vi "Motor Control NO PID AE Ver.vi"(0 "Direction":T2, 1 "AE Mode":T1, 2 "Speed":dbl, 3 "error in (no error)":errorcluster, 4 "Yaw":dbl) -> (5 "Speed & distance":T3, 6 "error out":errorcluster)   [LabVIEW 2018]
uses:
  MOTOR CONTROL NO PID AE DIRECTIONS type def.ctl
  MOTOR CONTROL NO PID AE DATA ENTRY MODE Type def.ctl
  <vilib>/Studica/Studica Toolkit/Background/Mxp Selection.ctl
panel:
  out "M2":dbl
  out "M1":dbl
  out "M0":dbl
  out "S2":dbl
  out "S1":dbl
  out "S0":dbl
  out "M2 Distance":dbl
  out "M1 Distance":dbl
  out "M0 Distance":dbl
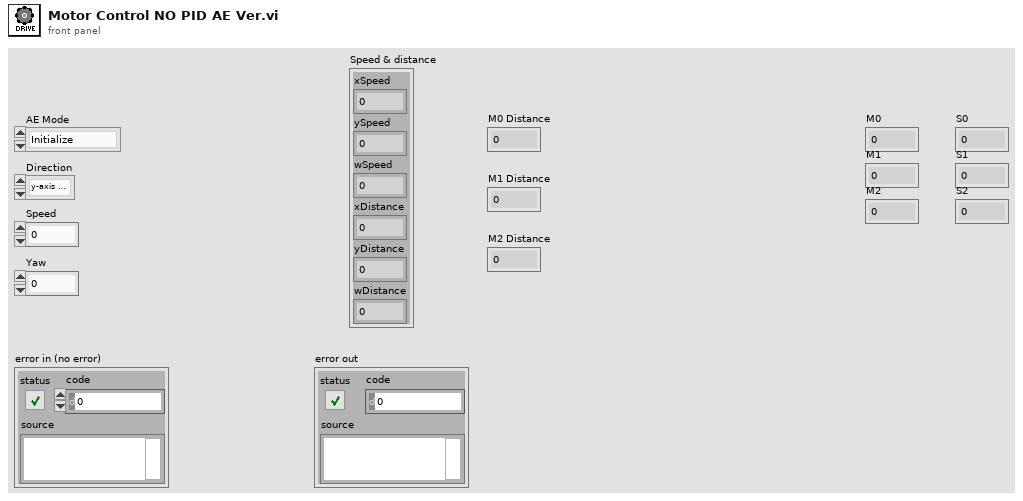
[diagram p1: front panel]
types:
  T1 = typedef "MOTOR CONTROL NO PID AE DATA ENTRY MODE Type def.ctl" = enum16{"Initialize", "Reset Encoders", "Write to motors", "Read from Encoders"}
  T2 = typedef "MOTOR CONTROL NO PID AE DIRECTIONS type def.ctl" = enum16{"y-axis movement", "x-axis movement", "Rotate", "Stop"}
  T3 = cluster{"xSpeed":dbl, "ySpeed":dbl, "wSpeed":dbl, "xDistance":dbl, "yDistance":dbl, "wDistance":dbl}
  T4 = typedef "Mxp Selection.ctl" = enum16{"MXP A", "MXP B"}
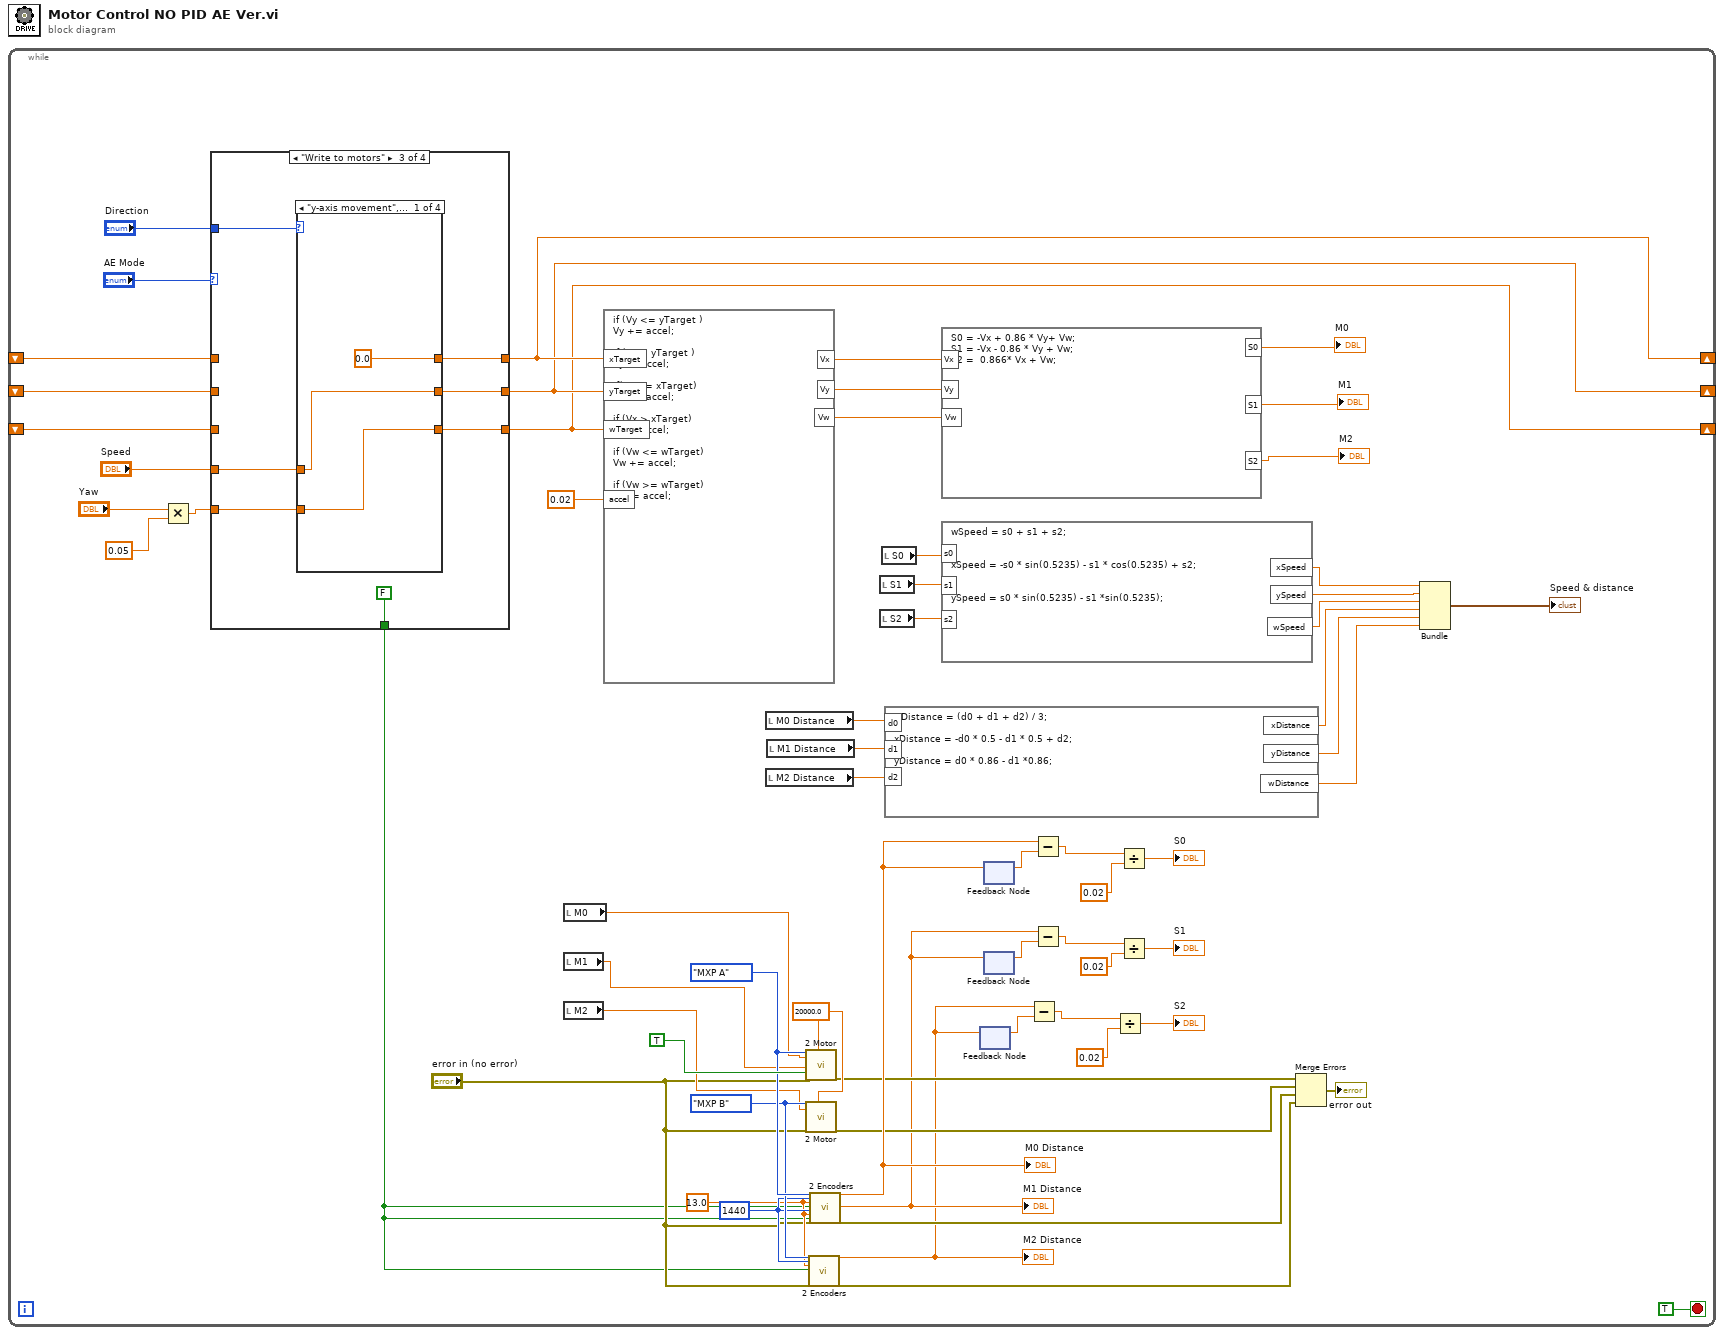
[diagram p0: block diagram]
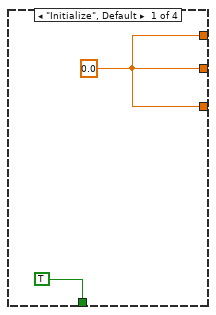
[diagram p2: hidden frame]
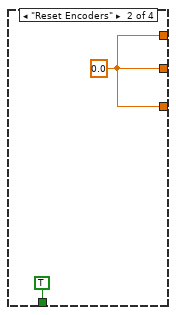
[diagram p3: hidden frame]
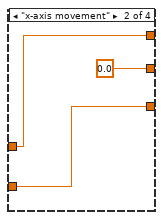
[diagram p4: hidden frame]
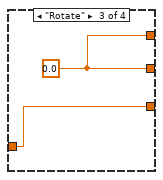
[diagram p5: hidden frame]
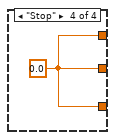
[diagram p6: hidden frame]
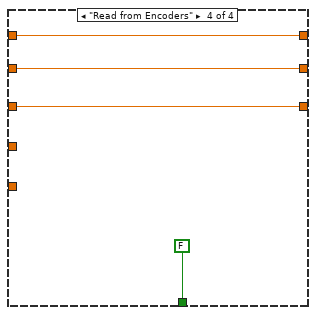
[diagram p7: hidden frame]
diagram:
  n1 = while {
    shift-right: [w11] -> _
    shift-left: _ -> [w7]
    shift-right: [w10] -> _
    shift-left: _ -> [w6]
    shift-right: [w9] -> _
    shift-left: _ -> [w5]
    stop <- TRUE stop-if-true
    w59 = 13.0 ("Wheel Diameter M0 (inches)")
    w60 = u32 1440 ("Ticks Per Rev M0")
    w64 = 20000.0 ("Frequency [Hz]")
    w62 = Mxp_Selection."MXP A" ("Mxp Side")
    w61 = Mxp_Selection."MXP B" ("Mxp Side")
    n2 = Multiply(x="Yaw", y=0.05) -> (x*y=w3:dbl)
    n3 = case shown="\"Write to motors\"" "AE Mode" {
      tunnel: "Direction" -> [_ _ w75 _]
      tunnel: "Speed" -> [_ _ w74 _]
      tunnel: w3 -> [_ _ w73 _]
      tunnel: [w66 w67 w72 w88] -> w11
      tunnel: [w66 w67 w71 w86] -> w9
      tunnel: [w66 w67 w70 w87] -> w10
      tunnel: w7 -> [_ _ _ w88]
      tunnel: w6 -> [_ _ _ w87]
      tunnel: w5 -> [_ _ _ w86]
      tunnel: [TRUE TRUE FALSE FALSE] -> w4
      frame "Initialize", Default {
        w66 = 0.0 ("input variable")
      }
      frame "Reset Encoders" {
        w67 = 0.0 ("input variable")
      }
      frame "Write to motors" {
        n4 = case shown="\"y-axis movement\", Default" w75 {
          tunnel: w74 -> [w78 w81 w83 _]
          tunnel: w73 -> [w77 w80 _ _]
          tunnel: [0.0 ("Speed") w81 w82 w84] -> w72
          tunnel: [w77 w80 w83 w84] -> w71
          tunnel: [w78 0.0 ("input variable") w82 w84] -> w70
          frame "y-axis movement", Default {
          }
          frame "x-axis movement" {
          }
          frame "Rotate" {
            w82 = 0.0 ("input variable")
          }
          frame "Stop" {
            w84 = 0.0 ("input variable")
          }
        }
      }
      frame "Read from Encoders" {
      }
    }
    n5 = local read "M0"() -> (w38:dbl)
    n6 = local read "M1"() -> (w37:dbl)
    n7 = local read "M2"() -> (w36:dbl)
    n8 = formula code="if (Vy <= yTarget )\nVy += accel;\n\nif (Vy > yTarget )\nVy -= accel;\n\nif(Vx <= xTarget)\nVx += accel;\n\nif (Vx > xTarget)\nVx -= accel;\n\nif (Vw <= wTarget)\nVw += accel;\n\nif (Vw >= wTarget)\nVw -= accel;"("xTarget"=w11, "yTarget"=w10, "wTarget"=w9, "accel"=0.02 ("input variable")) -> ("Vy"=w19:dbl, "Vx"=w20:dbl, "Vw"=w18:dbl)
    n9 = local read "M0 Distance"() -> (w32:dbl)
    n10 = local read "M2 Distance"() -> (w30:dbl)
    n11 = local read "M1 Distance"() -> (w31:dbl)
    n12 = call <vilib>:"2 Motor.vi"("Mxp Side"=w62, "Speed M0"=w38, "Speed M1"=w37, "Invert M1"=TRUE, "error in (no error)"="error in (no error)", "Frequency [Hz]"=w64) -> ("error out"=w54:errorcluster)  [unwired: 13 in]
    n13 = call <vilib>:"2 Motor.vi"("Mxp Side"=w61, "Speed M0"=w36, "error in (no error)"="error in (no error)", "Frequency [Hz]"=w64) -> ("error out"=w53:errorcluster)  [unwired: 15 in]
    n14 = call <vilib>:"2 Encoders.vi"("Mxp Side"=w61, "Ticks Per Rev M0"=w60, "Wheel Diameter M0 (inches)"=w59, "Reset Encoder 0"=w4, "error in (no error)"="error in (no error)") -> ("Distance M0 (inches)"=w42:dbl, "error out"=w51:errorcluster)  [unwired: 20 in, 1 out]
    "M2 Distance" <- w42
    n15 = call <vilib>:"2 Encoders.vi"("Mxp Side"=w62, "Ticks Per Rev M0"=w60, "Wheel Diameter M0 (inches)"=w59, "Reset Encoder 0"=w4, "Ticks Per Rev M1"=w60, "Wheel Diameter M1 (inches)"=w59, "Reset Encoder 1"=w4, "error in (no error)"="error in (no error)") -> ("Distance M0 (inches)"=w57:dbl, "Distance M1 (inches)"=w46:dbl, "error out"=w52:errorcluster)  [unwired: 17 in]
    "M0 Distance" <- w57
    "M1 Distance" <- w46
    n16 = local read "S1"() -> (w34:dbl)
    n17 = local read "S2"() -> (w33:dbl)
    n18 = local read "S0"() -> (w35:dbl)
    n19 = formula code="wDistance = (d0 + d1 + d2) / 3;\n\nxDistance = -d0 * 0.5 - d1 * 0.5 + d2;\n\nyDistance = d0 * 0.86 - d1 *0.86;"("d0"=w32, "d1"=w31, "d2"=w30) -> ("xDistance"=w25:dbl, "wDistance"=w23:dbl, "yDistance"=w24:dbl)
    n20 = formula code="S0 = -Vx + 0.86 * Vy+ Vw;\nS1 = -Vx - 0.86 * Vy + Vw;\nS2 =  0.866* Vx + Vw;"("Vx"=w20, "Vy"=w19, "Vw"=w18) -> ("S0"=→"M0":dbl, "S1"=→"M1":dbl, "S2"=→"M2":dbl)
    n21 = formula code="wSpeed = s0 + s1 + s2;\n\n\nxSpeed = -s0 * sin(0.5235) - s1 * cos(0.5235) + s2;\n\n\nySpeed = s0 * sin(0.5235) - s1 *sin(0.5235);"("s0"=w35, "s1"=w34, "s2"=w33) -> ("xSpeed"=w29:dbl, "ySpeed"=w28:dbl, "wSpeed"=w27:dbl)
    n22 = feedback #1() -> (w44:dbl)  [unwired: 1 in]
    n23 = feedback-in #1(w42) -> ()
    n24 = feedback #2() -> (w56:dbl)  [unwired: 1 in]
    n25 = feedback-in #2(w57) -> ()
    n26 = feedback #3() -> (w48:dbl)  [unwired: 1 in]
    n27 = feedback-in #3(w46) -> ()
    n28 = Subtract(x=w42, y=w44) -> (x-y=w45:dbl)
    n29 = Subtract(x=w57, y=w56) -> (x-y=w58:dbl)
    n30 = Subtract(x=w46, y=w48) -> (x-y=w49:dbl)
    n31 = Divide(x=w45, y=0.02) -> (x/y=→"S2":dbl)
    n32 = Divide(x=w58, y=0.02) -> (x/y=→"S0":dbl)
    n33 = Divide(x=w49, y=0.02) -> (x/y=→"S1":dbl)
    n34 = Merge Errors(w54, w53, w52, w51) -> (→"error out":errorcluster)
    n35 = Bundle("xSpeed"=w29, "ySpeed"=w28, "wSpeed"=w27, "xDistance"=w25, "yDistance"=w24, "wDistance"=w23) -> (→"Speed & distance":T3)  [unwired: 1 in]
  }
